vi "Validate Fixed Header.vi"(8 "error in (no error)":errorcluster, 11 "PUBREL in":refnum<class "PUBREL.lvclass">) -> (0 "error out":errorcluster, 1 "Valid":bool, 3 "PUBREL out":refnum<class "PUBREL.lvclass">)   [LabVIEW 2013, in "MQTT_Control_Packets.lvlib" / "PUBREL.lvclass"]
uses:
  PUBREL.lvclass
  ControlPacket/ControlPacket.lvclass/ControlPacket.ctl
  ControlPacket/ControlPacket.lvclass
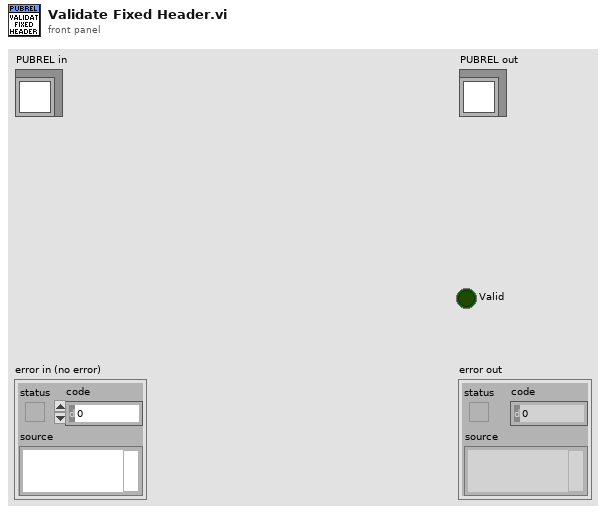
[diagram p1: front panel]
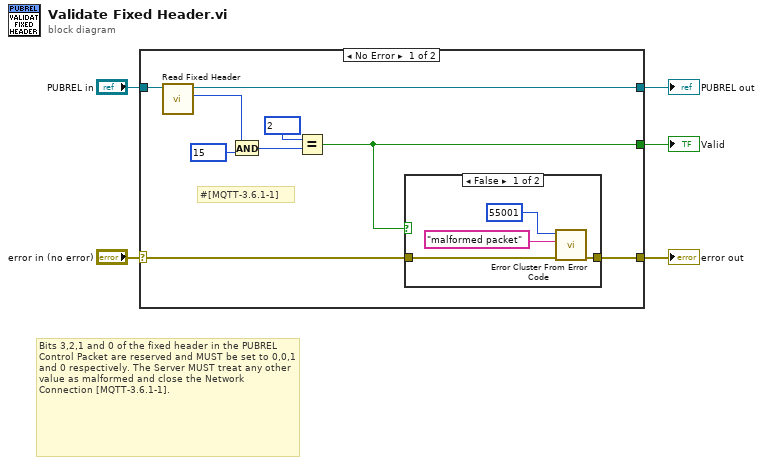
[diagram p0: block diagram]
diagram:
  # "Bits 3,2,1 and 0 of the fixed header in the PUBREL Control Packet are reserved and MUST be set to 0,0,1 and 0 respectively. The Server MUST treat any other value as malformed and close the Network Connection [MQTT-3.6.1-1]."
  n1 = case shown="No Error" "error in (no error)" {
    selector: "error in (no error)" -> [w9 w21]
    tunnel: [w8 w21] -> w5
    tunnel: [w6 _] -> w4
    tunnel: [w7 w20] -> w3
    tunnel: "PUBREL in" -> [w10 w20]
    frame No Error {
      # "#[MQTT-3.6.1-1]"
      n2 = call "Read Fixed Header.vi"("ControlPacket in"=w10) -> ("Fixed Header"=w13:u8, "ControlPacket out"=w7:refnum<class "PUBREL.lvclass">)  [unwired: 9 in]
      n3 = And(x=w13, y=u8 15) -> (x .and. y?=w12:u8)
      n4 = Equal?(x=u8 2 ("y"), y=w12) -> (x = y?=w6:bool)
      n5 = case shown="False" w6 {
        tunnel: [w16 w19] -> w8
        tunnel: w9 -> [w15 w19]
        frame False {
          n6 = call <vilib>:"Error Cluster From Error Code.vi"("error in (no error)"=w15, "error message (\"\")"="malformed packet" ("error message (\"\")"), "error code (0)"=55001) -> ("error out"=w16:errorcluster)  [unwired: 6 in]
        }
        frame True {
        }
      }
    }
    frame Error {
    }
  }
  "Valid" <- w4
  "error out" <- w5
  "PUBREL out" <- w3
